vi "Close Interface.vi"(8 "error in (no error)":errorcluster, 11 "Actor Interface in":refnum<data-value>) -> (0 "error out":errorcluster)   [LabVIEW 2018, in "Actor.lvlib" / "Actor-Interface.lvclass"]
uses:
  Actor-Interface.lvclass
  Actor-Interface.lvclass/Actor-Interface.ctl
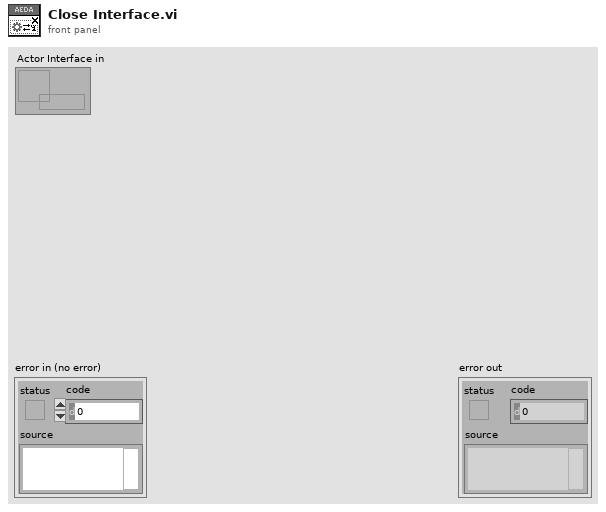
[diagram p1: front panel]
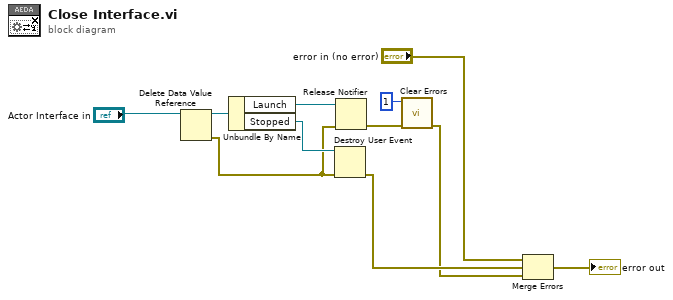
[diagram p0: block diagram]
diagram:
  n1 = Delete Data Value Reference(data value reference="Actor Interface in") -> (data value=w10:refnum<class "Actor-Interface.lvclass">, error out=w2:errorcluster)  [unwired: 1 in]
  n2 = Unbundle By Name(w10) -> ("Launch"=w9:refnum<notifier>, "Stopped"=w8:refnum<user-event>)
  n3 = Destroy User Event(user event=w8, error in=w2) -> (error out=w5:errorcluster)
  n4 = Release Notifier(notifier=w9, error in (no error)=w2) -> (error out=w7:errorcluster)  [unwired: 1 in, 2 out]
  n5 = call <vilib>:"Clear Errors.vi"("error in (no error)"=w7, "specific error code to clear (0: all)"=1) -> ("error out"=w4:errorcluster)  [unwired: 4 in, 1 out]
  n6 = Merge Errors("error in (no error)", w5, w4) -> (→"error out":errorcluster)
